vi "IsSearchGoalNode.vi"(8 "error in (no error)":errorcluster, 10 "NodeToIdentify in":refnum<data-value>, 11 "LinkedList in":refnum<class "LinkedList.lvclass">) -> (0 "error out":errorcluster, 1 "IsGoalNode":bool, 2 "NodeToIdentify out":refnum<data-value>, 3 "LinkedList out":refnum<class "LinkedList.lvclass">)   [LabVIEW 2013, in "LinkedList.lvclass"]
doc: "Abstract method. Override this VI to implement a search of a linked list. This VI is responsible for determining when we have found the node we are searching for."
uses:
  LinkedList.lvclass
  LLNode/LLNode.lvclass
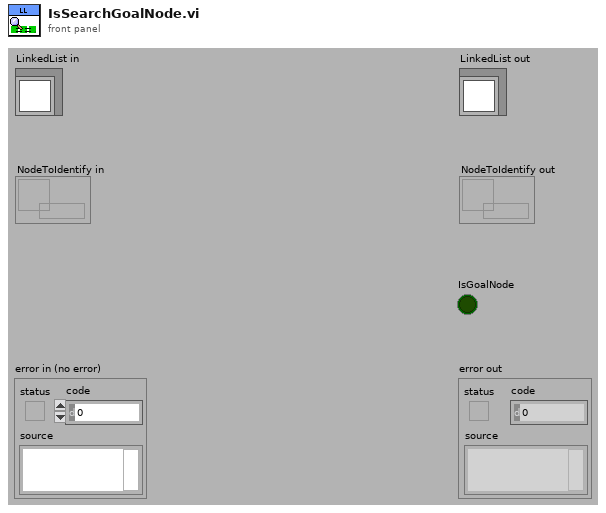
[diagram p1: front panel]
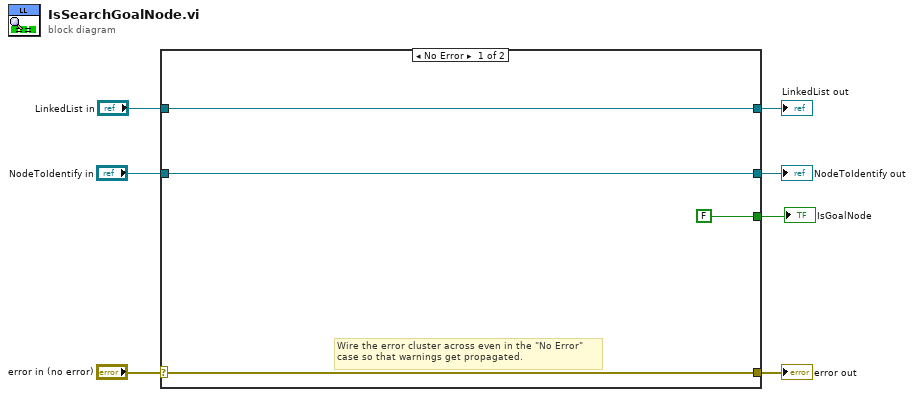
[diagram p0: block diagram]
diagram:
  n1 = case shown="No Error" "error in (no error)" {
    selector: "error in (no error)" -> [w11 w14]
    tunnel: [w11 w14] -> w6
    tunnel: [w10 w13] -> w4
    tunnel: "LinkedList in" -> [w10 w13]
    tunnel: "NodeToIdentify in" -> [w9 w12]
    tunnel: [w9 w12] -> w2
    tunnel: [FALSE _] -> w1
    frame No Error {
      # "Wire the error cluster across even in the \"No Error\"\ncase so that warnings get propagated."
    }
    frame Error {
    }
  }
  "error out" <- w6
  "LinkedList out" <- w4
  "NodeToIdentify out" <- w2
  "IsGoalNode" <- w1
